vi "UnInstall Script.vi"(8 "error in (no error)":errorcluster) -> (0 "error out":errorcluster)   [LabVIEW 2014]
panel:
  out "path":path
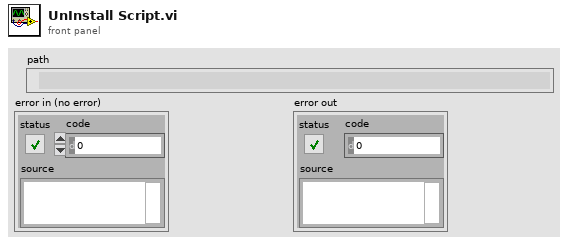
[diagram p1: front panel]
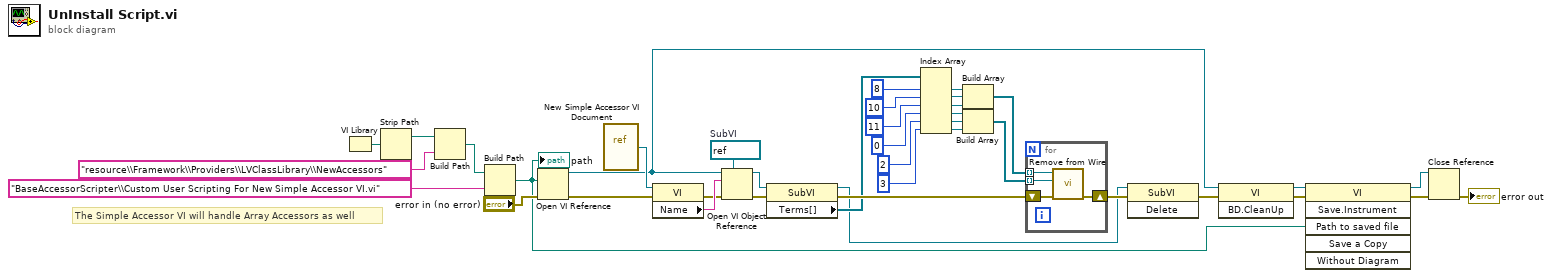
[diagram p0: block diagram]
diagram:
  w11 = refnum<vi> refnum  # SubVI
  # "The Simple Accessor VI will handle Array Accessors as well"
  n1 = VI Library() -> (path=w39:path)
  n2 = Strip Path(path=w39) -> (stripped path=w38:path)  [unwired: 1 out]
  n3 = Build Path(base path=w38, name or relative path="resource\\Framework\\Providers\\LVClassLibrary\\NewAccessors") -> (appended path=w36:path)
  n4 = Build Path(base path=w36, name or relative path="BaseAccessorScripter\\Custom User Scripting For New Simple Accessor VI.vi") -> (appended path=w1:path)
  "path" <- w1
  n5 = Open VI Reference(vi path=w1, error in (no error)="error in (no error)") -> (vi reference=w6:refnum<vi>, error out=w8:errorcluster)  [unwired: 4 in]
  n6 = vi-ref "New Simple Accessor VI Document.vi"() -> (w10:refnum<vi>)
  n7 = property class="VI"(reference=w10, error in=w8) -> (error out=w7:errorcluster, "Name"=w9:string)  [unwired: 1 out]
  n8 = Open VI Object Reference(7:w11, 8:w7, 10:w9, 11:w6) -> (0:w13:errorcluster, 3:w12:refnum<vi>)
  n9 = property class="SubVI"(reference=w12, error in=w13) -> (reference out=w14:refnum<vi>, error out=w28:errorcluster, "Terms[]"=w21:refnum<vi>[])
  n10 = Index Array(array=w21, index #1=8 ("index"), index #2=10 ("index"), index #3=11 ("index"), index #4=0 ("index"), index #5=2 ("index"), index #6=3 ("index")) -> (element #1=w32:refnum<vi>, element #2=w33:refnum<vi>, element #3=w34:refnum<vi>, element #4=w29:refnum<vi>, element #5=w30:refnum<vi>, element #6=w31:refnum<vi>)
  n11 = Build Array(w32, w33, w34) -> (w17:refnum<vi>[])
  n12 = Build Array(w29, w30, w31) -> (w18:refnum<vi>[])
  n13 = for {
    shift-right: [w42] -> w16
    shift-left: w28 -> [w43]
    tunnel: w17 -> [w40] mode=indexing
    tunnel: w18 -> [w41] mode=indexing
    n14 = call "Remove from Wire.vi"("error in (no error)"=w43, "Output Term"=w41, "Input Term"=w40) -> ("error out"=w42:errorcluster)  [unwired: 8 in]
  }
  n15 = invoke class="SubVI" method="Delete"(reference=w14, error in=w16) -> (error out=w15:errorcluster)  [unwired: 1 in, 2 out]
  n16 = invoke class="VI" method="BD.CleanUp"(reference=w6, error in=w15) -> (reference out=w5:refnum<vi>, error out=w4:errorcluster)  [unwired: 1 in, 1 out]
  n17 = invoke class="VI" method="Save.Instrument"(reference=w5, error in=w4, "Path to saved file"=w1) -> (reference out=w2:refnum<vi>, error out=w3:errorcluster)  [unwired: 3 in, 4 out]
  n18 = Close Reference(reference=w2, error in (no error)=w3) -> (error out=→"error out":errorcluster)
